vi "SetChainMask.vi"(8 "error in (no error)":errorcluster, 10 "ChainMask":u8 format="0x%02x", 11 "ControlState in":T1 {"ChainMask" format="0x%02x"}) -> (0 "error out":errorcluster, 3 "ControlState out":T1 {"ChainMask" format="0x%02x"})   [LabVIEW 2025, in "ArduinoSerialBling.lvlib"]
uses:
  ArduinoSerialBling.lvlib
  ControlState.ctl
  ConnectionType.ctl
  UdpConnection.ctl
  ChainState.ctl
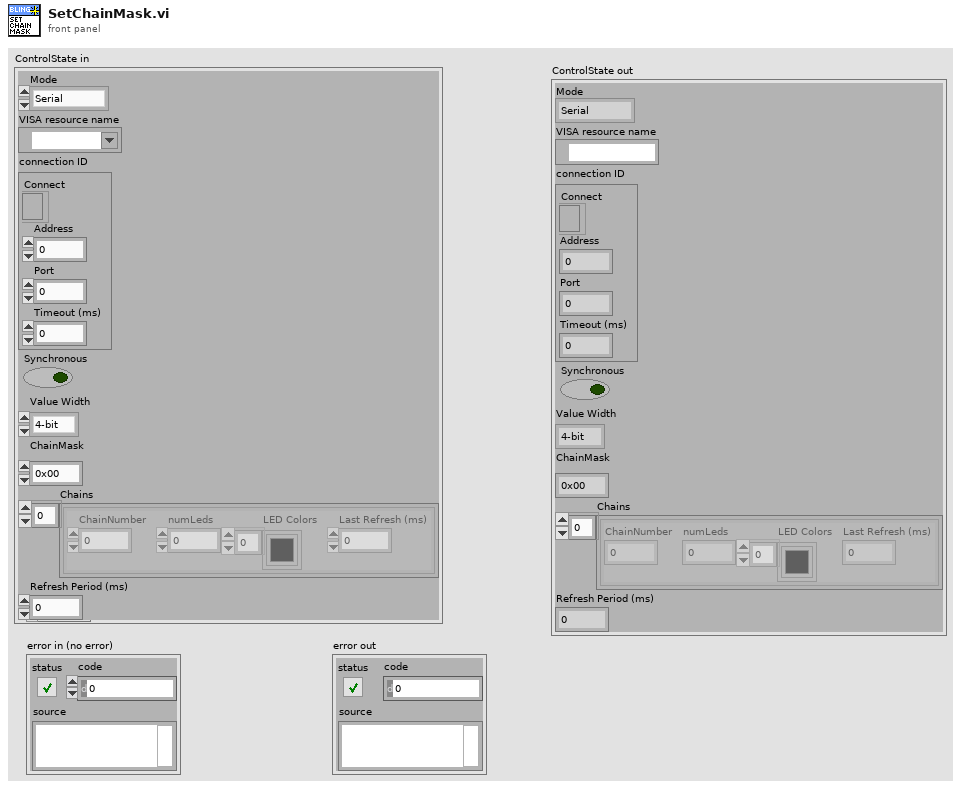
[diagram p1: front panel]
types:
  T1 = typedef "ArduinoSerialBling.lvlib/ControlState.ctl" = cluster{"Mode":T2, "VISA resource name":refnum<visa-resource-name>, "connection ID":T3, "Synchronous":bool, "Value Width":enum16{"4-bit", "8-bit"}, "ChainMask":u8, "Chains":T4[], "Refresh Period (ms)":u32}
  T2 = typedef "ConnectionType.ctl" = enum16{"Serial", "Ethernet", "Offline"}
  T3 = typedef "UdpConnection.ctl" = cluster{"Connect":refnum<k16>, "Address":u32, "Port":u16, "Timeout (ms)":i32}
  T4 = typedef "ArduinoSerialBling.lvlib/ChainState.ctl" = cluster{"ChainNumber":u8, "numLeds":u8, "LED Colors":u32[], "Last Refresh (ms)":u32}
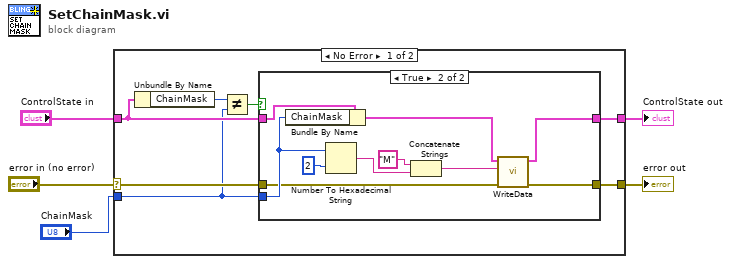
[diagram p0: block diagram]
diagram:
  n1 = case shown="No Error" "error in (no error)" {
    selector: "error in (no error)" -> [w12 w25]
    tunnel: "ControlState in" -> [w11 w26]
    tunnel: "ChainMask" -> [w8 _]
    tunnel: [w7 w25] -> w4
    tunnel: [w6 w26] -> w5
    frame No Error {
      n2 = Unbundle By Name(w11) -> ("ChainMask"=w10:u8)
      n3 = Not Equal?(x=w10, y=w8) -> (x != y?=w9:bool)
      n4 = case shown="True" w9 {
        tunnel: w12 -> [w13 w18]
        tunnel: w11 -> [w14 w20]
        tunnel: w8 -> [_ w23]
        tunnel: [w13 w17] -> w7
        tunnel: [w14 w19] -> w6
        frame False {
        }
        frame True {
          n5 = Bundle By Name(cluster=w20, "ChainMask"=w23) -> (w15:T1)
          n6 = Number To Hexadecimal String(1:i16 2 ("width (-)"), 2:w23) -> (0:w21:string)
          n7 = Concatenate Strings("M", w21) -> (w16:string)
          n8 = call "WriteData.vi"("error in (no error)"=w18, "Command"=w16, "ControlState in"=w15) -> ("error out"=w17:errorcluster, "ControlState out"=w19:T1)  [unwired: 5 in, 2 out]
        }
      }
    }
    frame Error {
    }
  }
  "ControlState out" <- w5
  "error out" <- w4
